vi "make plots_fits.vi"() -> ()   [LabVIEW 2016]
panel:
  out "display fit 2":cluster{dbl[], dbl[]}[](graph)
  out "v":dbl[](array[numeric])
  out "A":dbl[](array[numeric])
  out "w":dbl
  in  "display fit":cluster{dbl[], dbl[]}[](graph)
  in  "Display best fit parameters":dbl[](array[numeric])
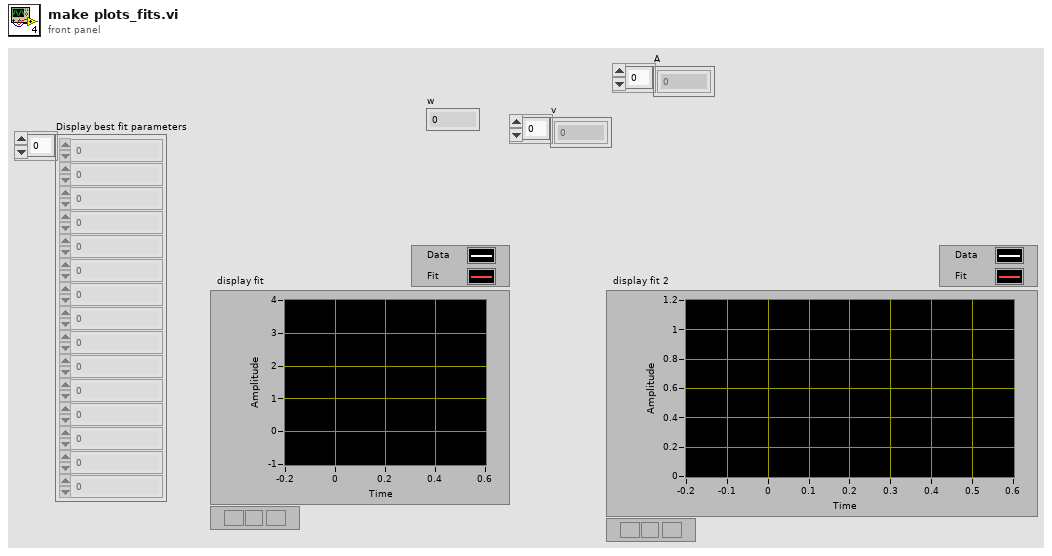
[diagram p1: front panel]
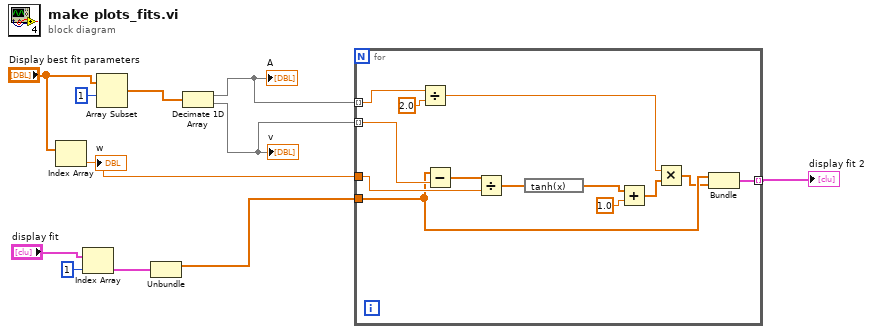
[diagram p0: block diagram]
diagram:
  n1 = Index Array(array="Display best fit parameters") -> (element=w6:dbl)  [unwired: 1 in]
  "w" <- w6
  n2 = Index Array(array="display fit", index=1) -> (element=w3:cluster{dbl[], dbl[]})
  n3 = Array Subset(array="Display best fit parameters", index=1) -> (w9:dbl[])  [unwired: 1 in]
  n4 = Unbundle(w3) -> (w2:dbl[])  [unwired: 1 out]
  n5 = Decimate 1D Array(w9) -> (w8:dbl[], w7:dbl[])
  "A" <- w8
  "v" <- w7
  n6 = for {
    tunnel: w8 -> [w24] mode=indexing
    tunnel: w7 -> [w22] mode=indexing
    tunnel: w6 -> [w20]
    tunnel: w2 -> [w13]
    tunnel: [w14] -> w1 mode=indexing
    n7 = Divide(x=w24, y=2.0) -> (x/y=w15:dbl)
    n8 = Subtract(x=w13, y=w22) -> (x-y=w21:dbl[])
    n9 = Divide(x=w21, y=w20) -> (x/y=w19:dbl[])
    n10 = expression code="tanh(x)"(w19) -> (w18:dbl[])
    n11 = Add(x=w18, y=1.0) -> (x+y=w16:dbl[])
    n12 = Multiply(x=w15, y=w16) -> (x*y=w12:dbl[])
    n13 = Bundle(w13, w12) -> (w14:cluster{dbl[], dbl[]})  [unwired: 1 in]
  }
  "display fit 2" <- w1
